vi "Set_Items.Listbox.vi"(8 "error in (no error)":errorcluster, 9 "Strings Array In (1D)":string[](array[string]), 10 "Listbox Name In":string, 11 "Data Value Reference in":T1) -> (0 "error out":errorcluster, 2 "reference out":refnum<vi>, 3 "Data Value Reference out":T1)   [LabVIEW 2020, in "CtlReferences.lvlib" / "CtlReferences.lvclass"]
uses:
  CtlReferences.lvclass
  TypeDefs/CtlLookup.ctl
  CtlReferences.lvclass/CtlReferences.ctl
  GetControlRef/GetControl_ListBox.vi
  GetControlRef/GetCtlRef_Wrap.vi
  GetCtlRef.vi
  <vilib>/Utility/error.llb/Error Cluster From Error Code.vi
  Error_ToSpecificClass.vi
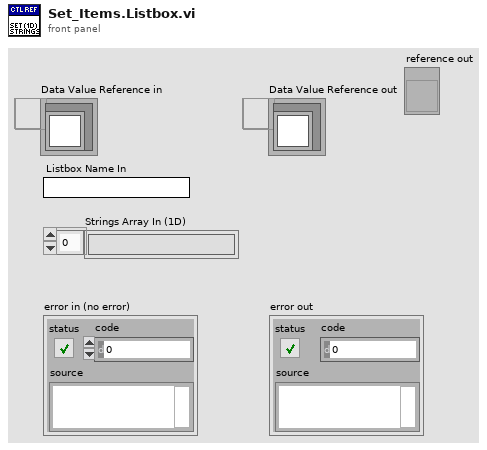
[diagram p1: front panel]
types:
  T1 = typedef "CtlReferences.lvlib/CtlReferences.lvclass/CtlLookup.ctl" = refnum<data-value>
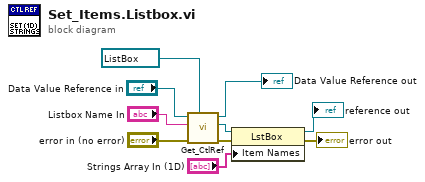
[diagram p0: block diagram]
diagram:
  n1 = call-poly "Get_CtlRef.vi"("Control Class"=refnum<vi> refnum, "error in (no error)"="error in (no error)", "Control Label"="Listbox Name In", "CtlLookup In"="Data Value Reference in") -> ("error out"=w6:errorcluster, "Reference Out"=w7:refnum<vi>, "CtlLookup Out"=→"Data Value Reference out":T1)  [unwired: 5 in]
  n2 = property class="LstBox"(reference=w7, error in=w6, "Item Names"="Strings Array In (1D)") -> (reference out=→"reference out":refnum<vi>, error out=→"error out":errorcluster)
